vi "Record data and move.vi"(0 "Lock in Input":T1, 1 "error in (no error)":errorcluster, 2 "Deceleration":bool, 5 "RESET":bool, 6 "Accelaration":bool, 7 "B axis":i32, 8 "Stop":bool, 9 "A axis":i32, 10 "Comport":refnum<visa-resource-name>="COM4") -> (3 "A out":dbl, 4 "VISA resource name out":refnum<visa-resource-name>)   [LabVIEW 2020]
uses:
  <vilib>/Instr/_visa.llb/VISA Configure Serial Port (Instr).vi
  Dependencies/Holmarc/2 axis linear/GlobalValue.vi
  <vilib>/Utility/file.llb/Write Delimited Spreadsheet (DBL).vi
  Dependencies/Stanford Research 830/Stanford Research 830.lvlib
panel:
  out "Output Graph":sgl[](graph)
  out "error out 2":errorcluster
  out "B out":dbl
  # "Configure Stage"
  # "COMPORT"
  # "To Move"
  # "Moved"
  # "Microns"
  # "Microns"
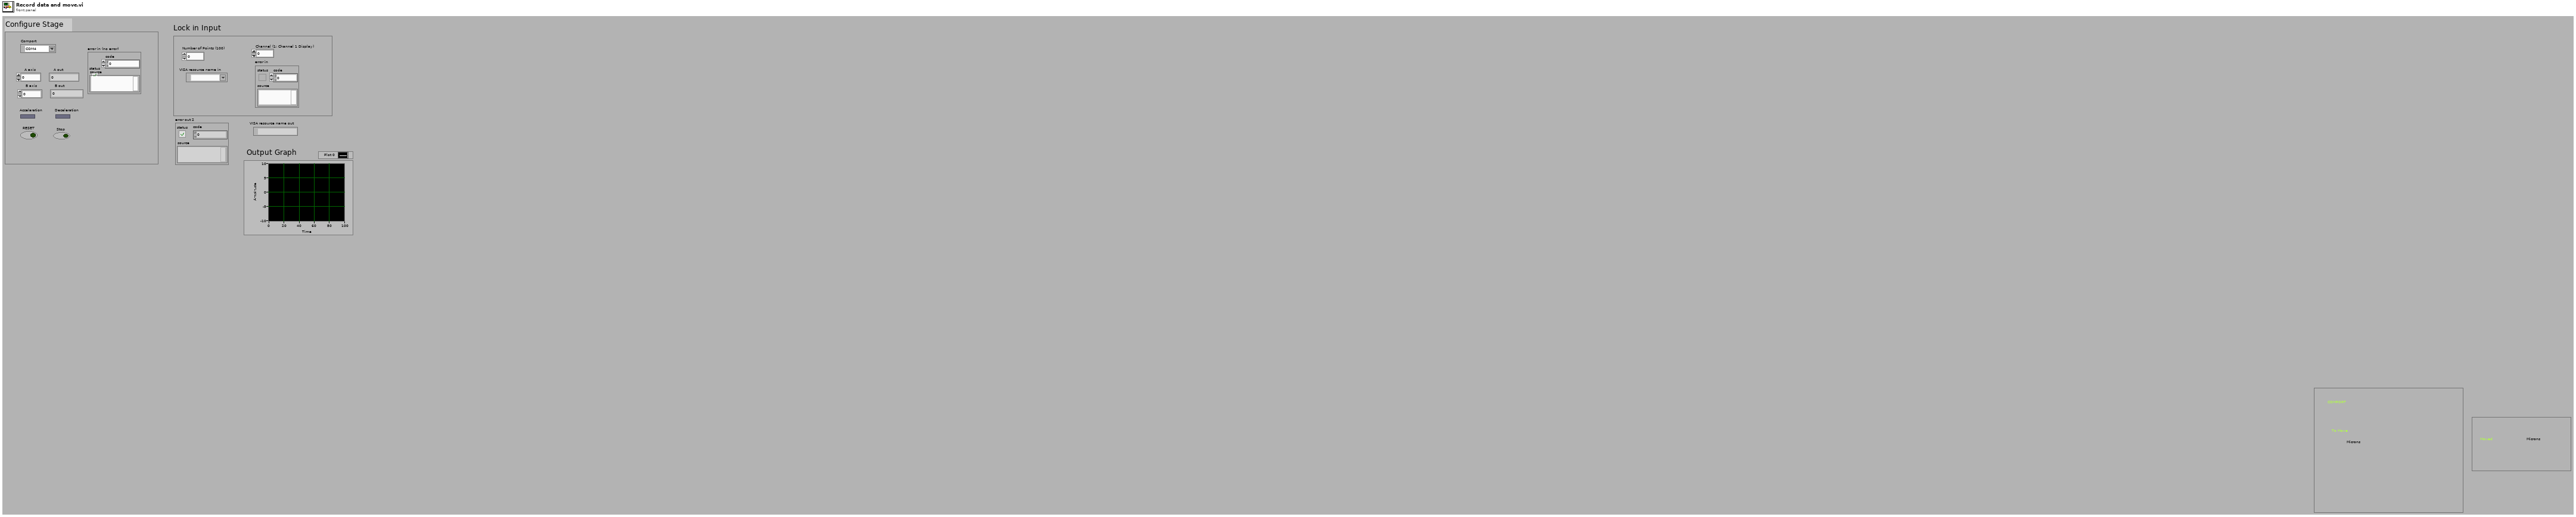
[diagram p1: front panel]
types:
  T1 = cluster{"Number of Points (100)":u32, "VISA resource name in":refnum<visa-resource-name>, "Channel (1: Channel 1 Display)":u16, "error in":errorcluster}
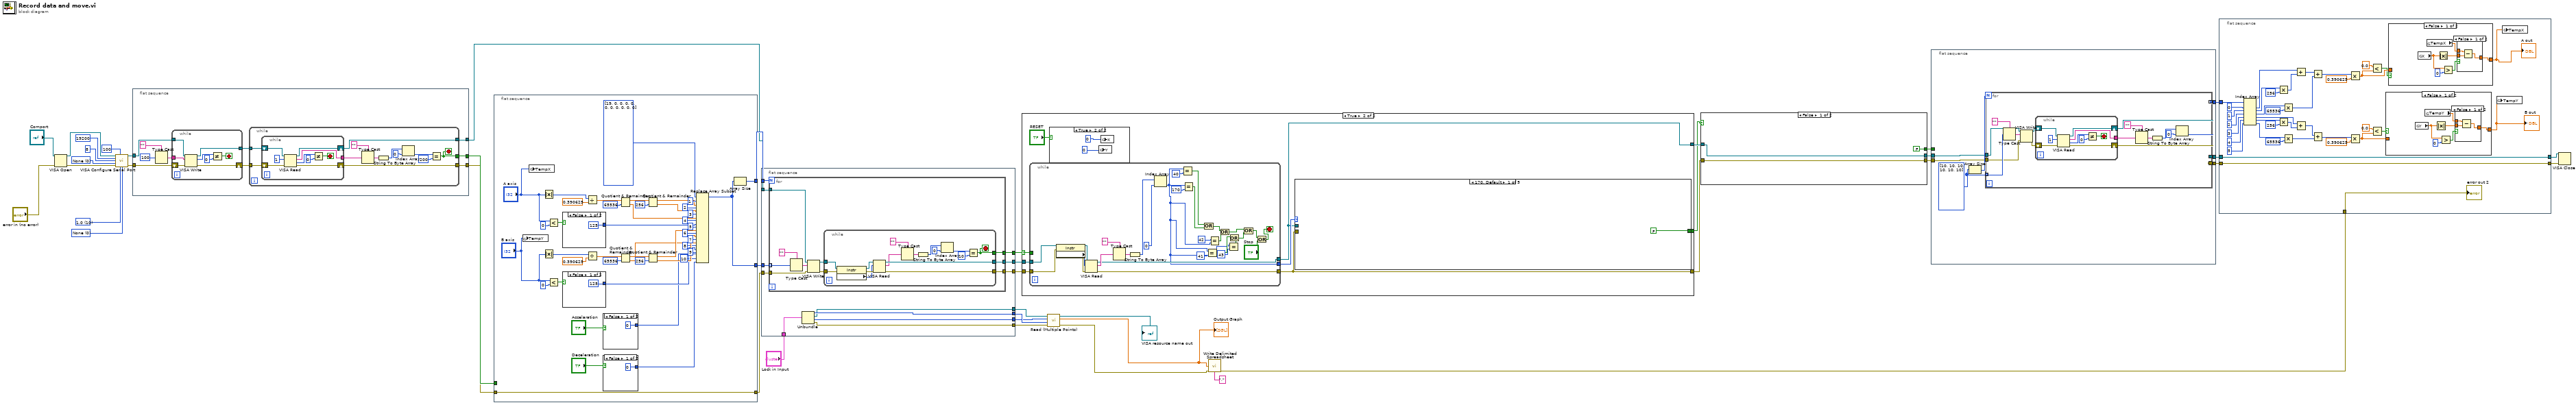
[diagram p0: block diagram]
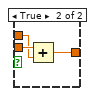
[diagram p2: hidden frame]
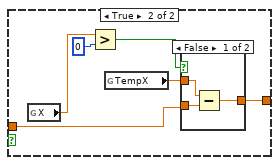
[diagram p3: hidden frame]
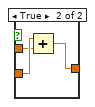
[diagram p4: hidden frame]
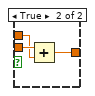
[diagram p5: hidden frame]
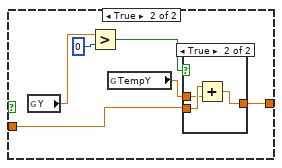
[diagram p6: hidden frame]
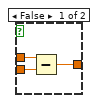
[diagram p7: hidden frame]
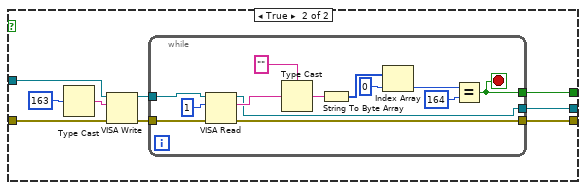
[diagram p8: hidden frame]
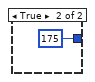
[diagram p9: hidden frame]
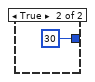
[diagram p10: hidden frame]
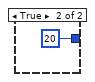
[diagram p11: hidden frame]
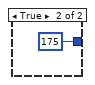
[diagram p12: hidden frame]
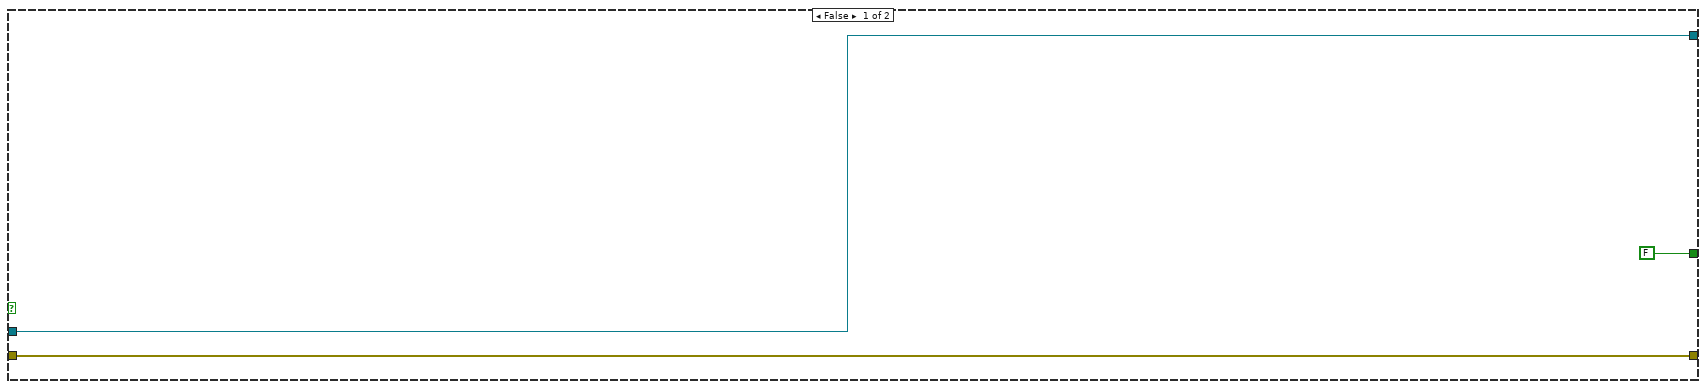
[diagram p13: hidden frame]
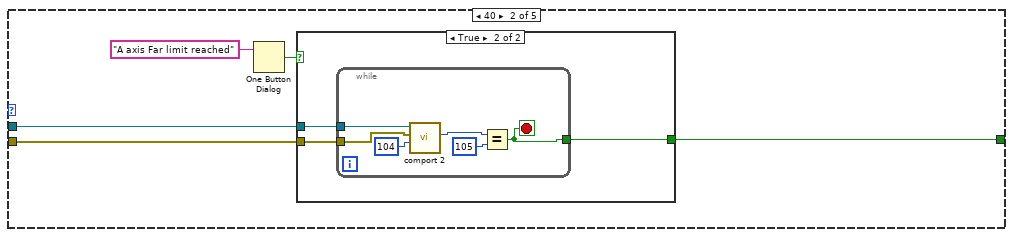
[diagram p15: hidden frame]
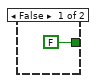
[diagram p16: hidden frame]
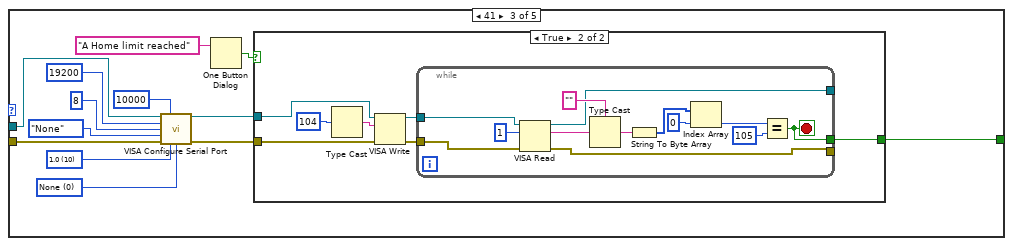
[diagram p17: hidden frame]
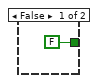
[diagram p18: hidden frame]
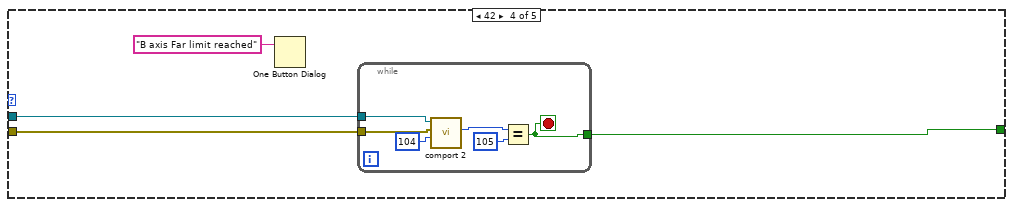
[diagram p19: hidden frame]
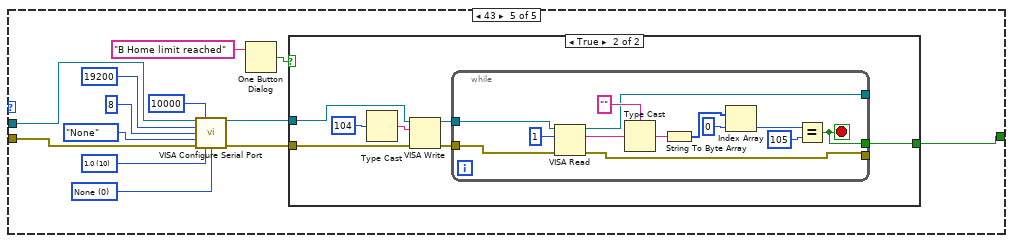
[diagram p20: hidden frame]
diagram:
  w37 = u16 0 items=["None"=0, "XON/XOFF"=1, "RTS/CTS"=2, "DTR/DSR"=4] ("flow control")
  w36 = u16 10 items=["1.0"=10, "1.5"=15, "2.0"=20] ("stop bits")
  w35 = u16 0 items=["None", "Odd", "Even", "Mark", "Space"] ("parity")
  n1 = VISA Open(error in (no error)="error in (no error)", VISA resource name="Comport") -> (VISA resource name=w40:refnum<visa-resource-name>, error out=w41:errorcluster)  [unwired: 3 in]
  n2 = call-poly "VISA Configure Serial Port"("VISA resource name"=w40, "timeout (10sec)"=u32 100, "baud rate (9600)"=u32 19200 ("baud rate"), "data bits (8)"=u16 8 ("data bits"), "parity (0:none)"=w35, "error in (no error)"=w41, "stop bits (10: 1 bit)"=w36, "flow control (0:none)"=w37) -> ("VISA resource name out"=w32:refnum<visa-resource-name>, "error out"=w31:errorcluster)  [unwired: 1 in, 5 out]
  n3 = flat-sequence {
    tunnel: w32 -> [w52]
    tunnel: w31 -> [w51]
    tunnel: [w50] -> w29
    tunnel: [w49] -> w16
    tunnel: [w43] -> w17
    frame #0 {
      n4 = Type Cast(type="", x=u8 100) -> (*(type *) &x=w47:string)
      n5 = while {
        tunnel: w47 -> [w60]
        shift-right: [w56] -> w44
        shift-left: w51 -> [w58]
        tunnel: w52 -> [w59]
        tunnel: [w57] -> w45
        stop <- w53 stop-if-true
        n6 = VISA Write(VISA resource name=w59, write buffer=w60, error in (no error)=w58) -> (VISA resource name out=w57:refnum<visa-resource-name>, return count=w55:u32, error out=w56:errorcluster)
        n7 = Not Equal?(x=w55, y=u32 0) -> (x != y?=w53:bool)
      }
      n8 = while {
        tunnel: w44 -> [w71]
        tunnel: [w69] -> w49
        tunnel: w45 -> [w72]
        tunnel: [w70] -> w50
        tunnel: [w64] -> w43
        stop <- w64 stop-if-true
        n9 = while {
          tunnel: [w76] -> w63
          shift-right: [w79] -> w70
          shift-left: w72 -> [w81]
          shift-right: [w78] -> w69
          shift-left: w71 -> [w80]
          stop <- w73 stop-if-true
          n10 = VISA Read(VISA resource name=w81, byte count=u32 1, error in (no error)=w80) -> (VISA resource name out=w79:refnum<visa-resource-name>, read buffer=w76:string, return count=w74:u32, error out=w78:errorcluster)
          n11 = Not Equal?(x=w74, y=u32 0) -> (x != y?=w73:bool)
        }
        n12 = Type Cast(type="", x=w63) -> (*(type *) &x=w61:string)
        n13 = String To Byte Array(string=w61) -> (unsigned byte array=w68:u8[])
        n14 = Index Array(array=w68, index=0) -> (element=w66:u8)
        n15 = Equal?(x=w66, y=u8 200) -> (x = y?=w64:bool)
      }
    }
  }
  n16 = flat-sequence {
    tunnel: [w120] -> w30
    tunnel: [w82] -> w28
    tunnel: w17 -> [_]
    tunnel: w16 -> [w117]
    tunnel: [w117] -> w15
    frame #0 {
      n17 = global write "GlobalValue.vi" "TempY"("B axis") -> ()
      n18 = global write "GlobalValue.vi" "TempX"("A axis") -> ()
      n19 = Absolute Value(x="A axis") -> (abs(x)=w121:i32)
      n20 = Absolute Value(x="B axis") -> (abs(x)=w109:i32)
      n21 = Less?(x="A axis", y=0) -> (x < y?=w123:bool)
      n22 = Less?(x="B axis", y=0) -> (x < y?=w104:bool)
      n23 = case shown="False" w123 {
        tunnel: [u16 125 u16 175] -> w95
        frame False {
        }
        frame True {
        }
      }
      n24 = case shown="False" w104 {
        tunnel: [u16 125 u16 175] -> w87
        frame False {
        }
        frame True {
        }
      }
      n25 = Divide(x=w121, y=0.390625) -> (x/y=w116:dbl)
      n26 = Divide(x=w109, y=0.390625) -> (x/y=w108:dbl)
      n27 = case shown="False" "Accelaration" {
        tunnel: [0 20] -> w85
        frame False {
        }
        frame True {
        }
      }
      n28 = case shown="False" "Deceleration" {
        tunnel: [0 30] -> w83
        frame False {
        }
        frame True {
        }
      }
      n29 = Quotient & Remainder(x=w116, y=65536) -> (x-y*floor(x/y)=w114:dbl, floor(x/y)=w98:dbl)
      n30 = Quotient & Remainder(x=w108, y=65536) -> (x-y*floor(x/y)=w106:dbl, floor(x/y)=w89:dbl)
      n31 = Quotient & Remainder(x=w114, y=256) -> (x-y*floor(x/y)=w101:dbl, floor(x/y)=w100:dbl)
      n32 = Quotient & Remainder(x=w106, y=256) -> (x-y*floor(x/y)=w93:dbl, floor(x/y)=w91:dbl)
      n33 = Replace Array Subset(array=u8[] [19, 0, 0, 0, 0, 0, 0, 0, 0, 0, 0], new element #1=w101, index #1=1 ("index"), new element #2=w100, index #2=2 ("index"), new element #3=w98, index #3=3 ("index"), new element #4=w95, index #4=4 ("index"), new element #5=w93, index #5=5 ("index"), new element #6=w91, index #6=6 ("index"), new element #7=w89, index #7=7 ("index"), new element #8=w87, index #8=8 ("index"), new element #9=w85, index #9=9 ("index"), new element #10=w83, index #10=10 ("index")) -> (w82:u8[])
      n34 = Array Size(array=w82) -> (size(s)=w120:i32)
    }
  }
  n35 = flat-sequence {
    tunnel: w30 -> [w145]
    tunnel: w29 -> [w144]
    tunnel: w15 -> [w143]
    tunnel: w28 -> [w142]
    tunnel: [w141] -> w27
    tunnel: [w140] -> w14
    tunnel: [w139] -> w26
    tunnel: "Lock in Input" -> [w138]
    tunnel: [w137] -> w9
    tunnel: [w136] -> w8
    tunnel: [w135] -> w7
    tunnel: [w134] -> w6
    frame #0 {
      n36 = for {
        N: w145 -> [_]
        tunnel: [w150] -> w139
        tunnel: w144 -> [w154]
        tunnel: [w152] -> w141
        tunnel: w143 -> [w153]
        tunnel: [w151] -> w140
        tunnel: w142 -> [w147] mode=indexing
        n37 = Type Cast(type="", x=w147) -> (*(type *) &x=w146:string)
        n38 = VISA Write(VISA resource name=w154, write buffer=w146, error in (no error)=w153) -> (VISA resource name out=w149:refnum<visa-resource-name>, error out=w148:errorcluster)  [unwired: 1 out]
        n39 = while {
          tunnel: w148 -> [w159]
          tunnel: [w169] -> w151
          tunnel: w149 -> [w160]
          tunnel: [w170] -> w152
          tunnel: [w164] -> w150
          stop <- w164 stop-if-true
          n40 = property class="Instr"(reference=w160, error in=w159) -> (reference out=w158:refnum<visa-resource-name>, error out=w157:errorcluster, "Serial Settings:Number of Bytes at Serial Port"=w156:u32)
          n41 = VISA Read(VISA resource name=w158, byte count=w156, error in (no error)=w157) -> (VISA resource name out=w170:refnum<visa-resource-name>, read buffer=w163:string, error out=w169:errorcluster)  [unwired: 1 out]
          n42 = Type Cast(type="", x=w163) -> (*(type *) &x=w161:string)
          n43 = String To Byte Array(string=w161) -> (unsigned byte array=w168:u8[])
          n44 = Index Array(array=w168, index=0) -> (element=w166:u8)
          n45 = Equal?(x=w166, y=u8 10) -> (x = y?=w164:bool)
        }
      }
      n46 = Unbundle(w138) -> ("Number of Points (100)"=w136:u32, "VISA resource name in"=w134:refnum<visa-resource-name>, "Channel (1: Channel 1 Display)"=w135:u16, "error in"=w137:errorcluster)
    }
  }
  n47 = case shown="True" w26 {
    selector: w26 -> [_ w174]
    tunnel: w27 -> [w173 w178]
    tunnel: w14 -> [w172 w180]
    tunnel: [w173 w177] -> w25
    tunnel: [w172 w176] -> w24
    tunnel: [FALSE w175] -> w11
    frame False {
    }
    frame True {
      n48 = while {
        tunnel: w180 -> [w196]
        tunnel: [w200] -> w177
        tunnel: [w202] -> w176
        tunnel: [w182] -> w179
        tunnel: w178 -> [w197]
        tunnel: w174 -> [_]
        stop <- w183 stop-if-true
        n49 = property class="Instr"(reference=w197, error in=w196) -> (reference out=w195:refnum<visa-resource-name>, error out=w194:errorcluster, "Serial Settings:Number of Bytes at Serial Port"=w193:u32)
        n50 = VISA Read(VISA resource name=w195, byte count=w193, error in (no error)=w194) -> (VISA resource name out=w200:refnum<visa-resource-name>, read buffer=w209:string, error out=w202:errorcluster)  [unwired: 1 out]
        n51 = Type Cast(type="", x=w209) -> (*(type *) &x=w210:string)
        n52 = String To Byte Array(string=w210) -> (unsigned byte array=w208:u8[])
        n53 = Index Array(array=w208, index=0) -> (element=w182:u8)
        n54 = Equal?(x=w182, y=u8 40) -> (x = y?=w199:bool)
        n55 = Equal?(x=w182, y=u8 170) -> (x = y?=w201:bool)
        n56 = Or(x=w199, y=w201) -> (x .or. y?=w190:bool)
        n57 = Equal?(x=w182, y=u8 41) -> (x = y?=w188:bool)
        n58 = Equal?(x=u8 42 ("y"), y=w182) -> (x = y?=w189:bool)
        n59 = Or(x=w190, y=w189) -> (x .or. y?=w198:bool)
        n60 = Equal?(x=w182, y=u8 43) -> (x = y?=w187:bool)
        n61 = Or(x=w188, y=w187) -> (x .or. y?=w186:bool)
        n62 = Or(x=w198, y=w186) -> (x .or. y?=w185:bool)
        n63 = Or(x=w185, y="Stop") -> (x .or. y?=w183:bool)
      }
      n64 = case shown="True" "RESET" {
        frame False {
        }
        frame True {
          n65 = global write "GlobalValue.vi" "Y"(0) -> ()
          n66 = global write "GlobalValue.vi" "X"(0) -> ()
        }
      }
      n67 = case shown="170, Default" w179 {
        tunnel: w177 -> [_ w215 w238 w265 w275]
        tunnel: w176 -> [_ w216 w235 w264 w274]
        tunnel: [FALSE w214 w239 w263 w273] -> w175
        frame 170, Default {
        }
        frame 40 {
          n68 = One Button Dialog(message="A axis Far limit reached") -> (true=w217:bool)  [unwired: 1 in]
          n69 = case shown="True" w217 {
            tunnel: w216 -> [_ w221]
            tunnel: w215 -> [_ w222]
            tunnel: [FALSE w220] -> w214
            frame False {
            }
            frame True {
              n70 = while {
                tunnel: w222 -> [w228]
                tunnel: w221 -> [w227]
                tunnel: [w223] -> w220
                stop <- w223 stop-if-true
                n71 = call "comport 2.vi"("x"=u8 104, "error in (no error)"=w227, "VISA resource name"=w228) -> ("Numeric"=w225:u8)  [unwired: 6 in, 2 out]
                n72 = Equal?(x=w225, y=u8 105) -> (x = y?=w223:bool)
              }
            }
          }
        }
        frame 41 {
          w230 = u16 0 items=["None", "XON/XOFF", "RTS/CTS", "XON/XOFF & RTS/CTS", "DTR/DSR", "XON/XOFF & DTR/DSR"] ("flow control (0:none)")
          w231 = u16 10 items=["1.0"=10, "1.5"=15, "2.0"=20] ("stop bits (10: 1 bit)")
          n73 = call-poly "VISA Configure Serial Port"("VISA resource name"=w238, "timeout (10sec)"=u32 10000, "baud rate (9600)"=u32 19200, "data bits (8)"=u16 8, "parity (0:none)"=enum16{"None", "Odd", "Even", "Mark", "Space"}."None", "error in (no error)"=w235, "stop bits (10: 1 bit)"=w231, "flow control (0:none)"=w230) -> ("VISA resource name out"=w237:refnum<visa-resource-name>, "error out"=w236:errorcluster)  [unwired: 6 in]
          n74 = One Button Dialog(message="A Home limit reached") -> (true=w240:bool)  [unwired: 1 in]
          n75 = case shown="True" w240 {
            tunnel: w237 -> [_ w246]
            tunnel: w236 -> [_ w245]
            tunnel: [FALSE w243] -> w239
            frame False {
            }
            frame True {
              n76 = Type Cast(x=104) -> (*(type *) &x=w249:string)  [unwired: 1 in]
              n77 = VISA Write(VISA resource name=w246, write buffer=w249, error in (no error)=w245) -> (VISA resource name out=w247:refnum<visa-resource-name>, error out=w248:errorcluster)  [unwired: 1 out]
              n78 = while {
                tunnel: w248 -> [w262]
                tunnel: [w252] -> _
                tunnel: w247 -> [w261]
                tunnel: [w251] -> _
                tunnel: [w250] -> w243
                stop <- w250 stop-if-true
                n79 = VISA Read(VISA resource name=w261, byte count=u32 1, error in (no error)=w262) -> (VISA resource name out=w251:refnum<visa-resource-name>, read buffer=w253:string, error out=w252:errorcluster)  [unwired: 1 out]
                n80 = Type Cast(type="", x=w253) -> (*(type *) &x=w254:string)
                n81 = String To Byte Array(string=w254) -> (unsigned byte array=w258:u8[])
                n82 = Index Array(array=w258, index=0) -> (element=w255:u8)
                n83 = Equal?(x=w255, y=u8 105) -> (x = y?=w250:bool)
              }
            }
          }
        }
        frame 42 {
          n84 = One Button Dialog(message="B axis Far limit reached") -> ()  [unwired: 1 in, 1 out]
          n85 = while {
            tunnel: [w269] -> w263
            tunnel: w265 -> [w268]
            tunnel: w264 -> [w267]
            stop <- w269 stop-if-true
            n86 = call "comport 2.vi"("x"=u8 104, "error in (no error)"=w267, "VISA resource name"=w268) -> ("Numeric"=w271:u8)  [unwired: 6 in, 2 out]
            n87 = Equal?(x=w271, y=u8 105) -> (x = y?=w269:bool)
          }
        }
        frame 43 {
          w277 = u16 0 items=["None", "XON/XOFF", "RTS/CTS", "XON/XOFF & RTS/CTS", "DTR/DSR", "XON/XOFF & DTR/DSR"] ("flow control (0:none)")
          w278 = u16 10 items=["1.0"=10, "1.5"=15, "2.0"=20] ("stop bits (10: 1 bit)")
          n88 = call-poly "VISA Configure Serial Port"("VISA resource name"=w275, "timeout (10sec)"=u32 10000, "baud rate (9600)"=u32 19200, "data bits (8)"=u16 8, "parity (0:none)"=enum16{"None", "Odd", "Even", "Mark", "Space"}."None", "error in (no error)"=w274, "stop bits (10: 1 bit)"=w278, "flow control (0:none)"=w277) -> ("VISA resource name out"=w283:refnum<visa-resource-name>, "error out"=w282:errorcluster)  [unwired: 6 in]
          n89 = One Button Dialog(message="B Home limit reached") -> (true=w284:bool)  [unwired: 1 in]
          n90 = case shown="True" w284 {
            tunnel: w283 -> [_ w290]
            tunnel: w282 -> [_ w289]
            tunnel: [FALSE w287] -> w273
            frame False {
            }
            frame True {
              n91 = Type Cast(x=104) -> (*(type *) &x=w293:string)  [unwired: 1 in]
              n92 = VISA Write(VISA resource name=w290, write buffer=w293, error in (no error)=w289) -> (VISA resource name out=w291:refnum<visa-resource-name>, error out=w292:errorcluster)  [unwired: 1 out]
              n93 = while {
                tunnel: w292 -> [w306]
                tunnel: [w296] -> _
                tunnel: w291 -> [w305]
                tunnel: [w295] -> _
                tunnel: [w294] -> w287
                stop <- w294 stop-if-true
                n94 = VISA Read(VISA resource name=w305, byte count=u32 1, error in (no error)=w306) -> (VISA resource name out=w295:refnum<visa-resource-name>, read buffer=w297:string, error out=w296:errorcluster)  [unwired: 1 out]
                n95 = Type Cast(type="", x=w297) -> (*(type *) &x=w298:string)
                n96 = String To Byte Array(string=w298) -> (unsigned byte array=w302:u8[])
                n97 = Index Array(array=w302, index=0) -> (element=w299:u8)
                n98 = Equal?(x=w299, y=u8 105) -> (x = y?=w294:bool)
              }
            }
          }
        }
      }
    }
  }
  n99 = call "Read (Multiple Points).vi"("error in (no error)"=w9, "Number of Points (100)"=w8, "Channel (1: Channel 1 Display)"=w7, "VISA resource name"=w6) -> ("error out"=w4:errorcluster, "Measurements"=w1:sgl[], "VISA resource name out"=→"VISA resource name out":refnum<visa-resource-name>)  [unwired: 5 in]
  "Output Graph" <- w1
  n100 = call-poly <vilib>:"Write Delimited Spreadsheet.vi"("1D data"=w1, "error in (no error)"=w4, "delimiter (\\t)"="," ("delimiter (\\t)")) -> ("error out"=w2:errorcluster)  [unwired: 11 in, 1 out]
  n101 = case shown="False" w11 {
    tunnel: w25 -> [w309 w315]
    tunnel: w24 -> [w308 w314]
    tunnel: [FALSE w313] -> w18
    tunnel: [w309 w311] -> w23
    tunnel: [w308 w312] -> w22
    frame False {
    }
    frame True {
      n102 = Type Cast(x=163) -> (*(type *) &x=w318:string)  [unwired: 1 in]
      n103 = VISA Write(VISA resource name=w315, write buffer=w318, error in (no error)=w314) -> (VISA resource name out=w316:refnum<visa-resource-name>, error out=w317:errorcluster)  [unwired: 1 out]
      n104 = while {
        tunnel: w317 -> [w331]
        tunnel: [w321] -> w312
        tunnel: w316 -> [w330]
        tunnel: [w320] -> w313
        tunnel: [w319] -> w311
        stop <- w320 stop-if-true
        n105 = VISA Read(VISA resource name=w330, byte count=u32 1, error in (no error)=w331) -> (VISA resource name out=w319:refnum<visa-resource-name>, read buffer=w322:string, error out=w321:errorcluster)  [unwired: 1 out]
        n106 = Type Cast(type="", x=w322) -> (*(type *) &x=w323:string)
        n107 = String To Byte Array(string=w323) -> (unsigned byte array=w327:u8[])
        n108 = Index Array(array=w327, index=0) -> (element=w324:u8)
        n109 = Equal?(x=w324, y=u8 164) -> (x = y?=w320:bool)
      }
    }
  }
  n110 = flat-sequence {
    tunnel: w22 -> [w337]
    tunnel: [w335] -> w20
    tunnel: [w336] -> w21
    tunnel: w23 -> [w334]
    tunnel: [w333] -> w19
    tunnel: w18 -> [_]
    frame #0 {
      w332 = u8[] [10, 10, 10, 10, 10, 10]
      n111 = Array Size(array=w332) -> (size(s)=w338:i32)
      n112 = for {
        N: w338 -> [_]
        tunnel: w337 -> [w341]
        tunnel: [w348] -> w336
        tunnel: w334 -> [w342]
        tunnel: [w347] -> w335
        tunnel: [w346] -> w333 mode=indexing
        tunnel: w332 -> [w343] mode=indexing
        n113 = Type Cast(type="", x=w343) -> (*(type *) &x=w344:string)
        n114 = VISA Write(VISA resource name=w342, write buffer=w344, error in (no error)=w341) -> (VISA resource name out=w340:refnum<visa-resource-name>, error out=w339:errorcluster)  [unwired: 1 out]
        n115 = while {
          tunnel: [w357] -> w351
          shift-right: [w360] -> w348
          shift-left: w340 -> [w362]
          shift-right: [w359] -> w347
          shift-left: w339 -> [w361]
          stop <- w354 stop-if-true
          n116 = VISA Read(VISA resource name=w362, byte count=u32 1, error in (no error)=w361) -> (VISA resource name out=w360:refnum<visa-resource-name>, read buffer=w357:string, return count=w355:u32, error out=w359:errorcluster)
          n117 = Not Equal?(x=w355, y=u32 0) -> (x != y?=w354:bool)
        }
        n118 = Type Cast(type="", x=w351) -> (*(type *) &x=w349:string)
        n119 = String To Byte Array(string=w349) -> (unsigned byte array=w353:u8[])
        n120 = Index Array(array=w353, index=0) -> (element=w346:u8)
      }
    }
  }
  n121 = flat-sequence {
    tunnel: w21 -> [w369]
    tunnel: w20 -> [w368]
    tunnel: w19 -> [w400]
    tunnel: [w369] -> w13
    tunnel: [w368] -> w12
    tunnel: w2 -> [w363]
    frame #0 {
      n122 = Index Array(array=w400, index #1=0 ("index"), index #2=1 ("index"), index #3=2 ("index"), index #4=3 ("index"), index #5=4 ("index"), index #6=5 ("index")) -> (element #1=w390:u8, element #2=w377:u8, element #3=w376:u8, element #4=w372:u8, element #5=w371:u8, element #6=w370:u8)
      n123 = Multiply(x=w377, y=u16 256) -> (x*y=w396:u16)
      n124 = Multiply(x=w371, y=u16 256) -> (x*y=w386:u16)
      n125 = Multiply(x=w376, y=u32 65536) -> (x*y=w395:u32)
      n126 = Multiply(x=w370, y=u32 65536) -> (x*y=w385:u32)
      n127 = Add(x=w390, y=w396) -> (x+y=w394:u16)
      n128 = Add(x=w372, y=w386) -> (x+y=w384:u16)
      n129 = Add(x=w394, y=w395) -> (x+y=w392:u32)
      n130 = Add(x=w384, y=w385) -> (x+y=w380:u32)
      n131 = Multiply(x=w392, y=0.390625) -> (x*y=w367:dbl)
      n132 = Multiply(x=w380, y=0.390625) -> (x*y=w381:dbl)
      n133 = Less?(x=0.0, y=w367) -> (x < y?=w364:bool)
      n134 = Less?(x=0.0, y=w381) -> (x < y?=w382:bool)
      n135 = case shown="False" w382 {
        tunnel: w381 -> [_ w437]
        tunnel: [w427 w439] -> w365
        frame False {
          n136 = global read "GlobalValue.vi" "Y"() -> (w426:dbl)
          n137 = global read "GlobalValue.vi" "TempY"() -> (w428:dbl)
          n138 = Absolute Value(x=w426) -> (abs(x)=w425:dbl)
          n139 = Greater?(x=w426, y=0) -> (0:w429:bool)
          n140 = case shown="False" w429 {
            tunnel: w425 -> [w432 w436]
            tunnel: w428 -> [w433 w435]
            tunnel: [w431 w434] -> w427
            frame False {
              n141 = Subtract(x=w433, y=w432) -> (x-y=w431:dbl)
            }
            frame True {
              n142 = Add(x=w436, y=w435) -> (x+y=w434:dbl)
            }
          }
        }
        frame True {
          n143 = global read "GlobalValue.vi" "Y"() -> (w438:dbl)
          n144 = Greater?(x=w438, y=0) -> (0:w441:bool)
          n145 = global read "GlobalValue.vi" "TempY"() -> (w440:dbl)
          n146 = case shown="True" w441 {
            tunnel: w437 -> [w444 w448]
            tunnel: w440 -> [w445 w447]
            tunnel: [w443 w446] -> w439
            frame False {
              n147 = Subtract(x=w445, y=w444) -> (x-y=w443:dbl)
            }
            frame True {
              n148 = Add(x=w448, y=w447) -> (x+y=w446:dbl)
            }
          }
        }
      }
      "B out" <- w365
      n149 = case shown="False" w364 {
        tunnel: w367 -> [_ w413]
        tunnel: [w403 w415] -> w366
        frame False {
          n150 = global read "GlobalValue.vi" "X"() -> (w402:dbl)
          n151 = global read "GlobalValue.vi" "TempX"() -> (w404:dbl)
          n152 = Absolute Value(x=w402) -> (abs(x)=w401:dbl)
          n153 = Greater?(x=w402, y=0) -> (0:w405:bool)
          n154 = case shown="False" w405 {
            tunnel: w401 -> [w408 w412]
            tunnel: w404 -> [w409 w411]
            tunnel: [w407 w410] -> w403
            frame False {
              n155 = Subtract(x=w409, y=w408) -> (x-y=w407:dbl)
            }
            frame True {
              n156 = Add(x=w412, y=w411) -> (x+y=w410:dbl)
            }
          }
        }
        frame True {
          n157 = global read "GlobalValue.vi" "X"() -> (w414:dbl)
          n158 = Greater?(x=w414, y=0) -> (0:w417:bool)
          n159 = global read "GlobalValue.vi" "TempX"() -> (w416:dbl)
          n160 = case shown="False" w417 {
            tunnel: w413 -> [w420 w424]
            tunnel: w416 -> [w421 w423]
            tunnel: [w419 w422] -> w415
            frame False {
              n161 = Subtract(x=w421, y=w420) -> (x-y=w419:dbl)
            }
            frame True {
              n162 = Add(x=w424, y=w423) -> (x+y=w422:dbl)
            }
          }
        }
      }
      "A out" <- w366
      n163 = global write "GlobalValue.vi" "TempY"(w365) -> ()
      n164 = global write "GlobalValue.vi" "TempX"(w366) -> ()
      "error out 2" <- w363
    }
  }
  n165 = VISA Close(VISA resource name=w13, error in (no error)=w12) -> ()  [unwired: 1 out]
